vi "Resolve Variant Task.vi"(10 "Value":dbl, 11 "Promise":refnum<class "Promise.lvclass">) -> ()   [LabVIEW 2020, in "Futures-Examples.lvlib"]
uses:
  Futures-Examples.lvlib
  Promises/Promise/Promise.lvclass
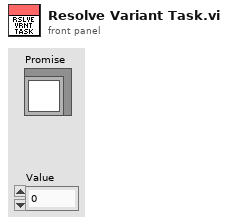
[diagram p1: front panel]
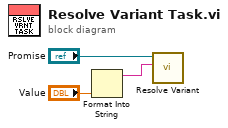
[diagram p0: block diagram]
diagram:
  n1 = Format Into String("Value") -> (resulting string=w1:string)  [unwired: 3 in, 1 out]
  n2 = call "Resolve Variant.vi"("Value"=w1, "Promise in"="Promise") -> ()  [unwired: 8 in, 2 out]
